vi "PQparameterStatus.vi"(7 "error in (no error)":errorcluster, 9 "paramName":string, 10 "conn":u64) -> (0 "error out":errorcluster, 2 "parameterstatus":string, 3 "conn_out":u64)   [LabVIEW 2019, in "libpqlv64.lvlib"]
doc: "Looks up a current parameter setting of the server.\n Certain parameter values are reported by the server automatically at connection startup or whenever their values change. PQparameterStatus can be used to interrogate these settings. It returns the current value of a parameter if known, or NULL if the parameter is not known.\n\nParameters reported as of the current release include server_version, server_encoding, client_encoding, is_superuser, session_authorization, DateStyle, TimeZone, integer_datetimes, and standard_conforming_strings. (server_encoding, TimeZone, and integer_datetimes were not reported by releases before 8.0; standard_conforming_strings was not reported by releases before 8.1.) Note that server_version, server_encoding and integer_datetimes cannot change after startup."
uses:
  libpqlv64.lvlib
  libpq.dll
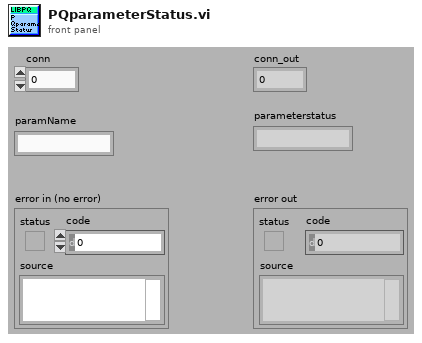
[diagram p1: front panel]
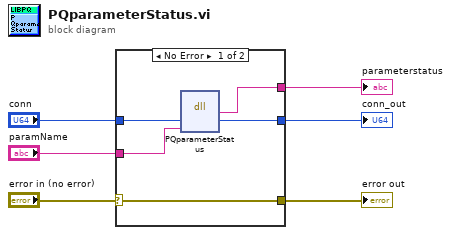
[diagram p0: block diagram]
diagram:
  n1 = case shown="No Error" "error in (no error)" {
    selector: "error in (no error)" -> [w11 w13]
    tunnel: [w11 w13] -> w5
    tunnel: [w10 _] -> w4
    tunnel: "paramName" -> [w9 _]
    tunnel: "conn" -> [w8 w12]
    tunnel: [w7 w12] -> w1
    frame No Error {
      n2 = dll-call lib="libpq.*" fn="PQparameterStatus"("conn"=w8, "paramName"=w9) -> ("parameterstatus"=w10:string, "conn"=w7:u64)  [unwired: 4 in, 2 out]
    }
    frame Error {
    }
  }
  "parameterstatus" <- w4
  "error out" <- w5
  "conn_out" <- w1
